vi "RunDevice.vi"() -> ()   [LabVIEW 2013]
uses:
  C:/Program Files/Newport/Piezo Motion Control/Newport AG-UC2-UC8 Applet/Samples/LabVIEW 2009/AgilisCmdLib.dll
  Program Files/Newport/Piezo Motion Control/Newport AG-UC2-UC8 Applet/Samples/LabVIEW 2009/AgilisCmdLib.dll
panel:
  in  "STOP":bool
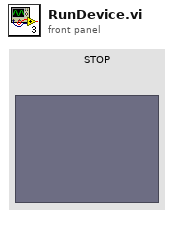
[diagram p1: front panel]
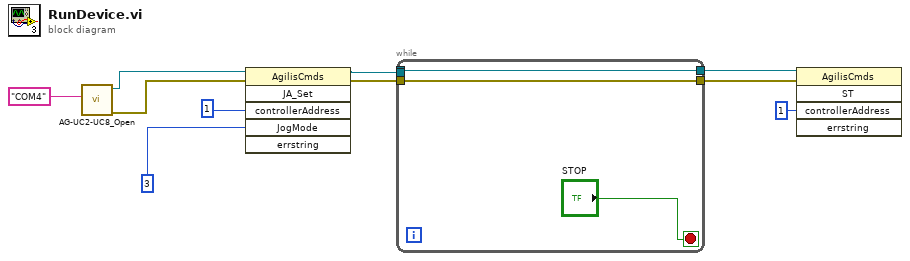
[diagram p0: block diagram]
diagram:
  n1 = call "AG-UC2-UC8_Open.vi"("Instrument Key IN"="COM4") -> ("error out"=w8:errorcluster, "AG-UC2-UC8 Reference"=w9:refnum<k24>)  [unwired: 3 in, 2 out]
  n2 = invoke class="AgilisCmds" method="JA_Set"(reference=w9, error in=w8, "controllerAddress"=1, "JogMode"=3) -> (reference out=w5:refnum<k24>, error out=w4:errorcluster)  [unwired: 2 in, 4 out]
  n3 = while {
    tunnel: [w13] -> _
    tunnel: w5 -> [w13]
    tunnel: w4 -> [w12]
    tunnel: [w13] -> w3
    tunnel: [w12] -> w2
    stop <- "STOP" stop-if-true
  }
  n4 = invoke class="AgilisCmds" method="ST"(reference=w3, error in=w2, "controllerAddress"=1) -> ()  [unwired: 2 in, 5 out]
